vi "CLSUIP_UnlockNewVI.vi"(8 "error in (no error)":errorcluster, 11 "VIRetooler":refnum<class "VIRetooler.lvclass">) -> (0 "error out":errorcluster)   [LabVIEW 2021, in "MemberVICreation.lvlib" / "VIRetooler.lvclass"]
uses:
  <resource>/Framework/Providers/LVClassLibrary/NewAccessors/VIRetooler/VIRetooler.lvclass
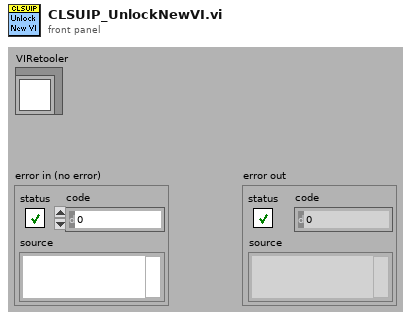
[diagram p1: front panel]
types:
  T1 = enum32{"invalid lock state", "Not Locked", "Locked (No Password)", "Password-protected"}
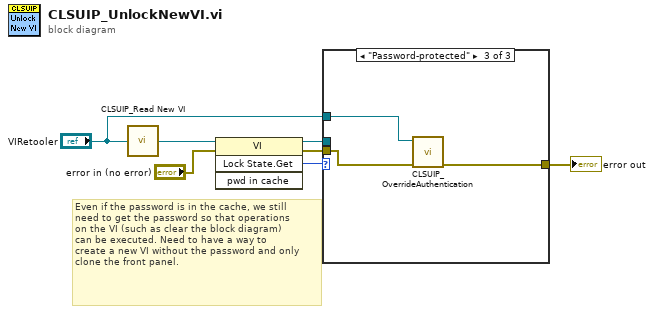
[diagram p0: block diagram]
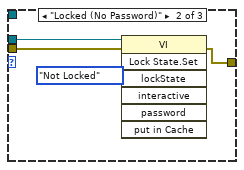
[diagram p3: hidden frame]
diagram:
  # "Even if the password is in the cache, we still\nneed to get the password so that operations\non the VI (such as clear the block diagram)\ncan be executed. Need to have a way to\ncreate a new VI without the password and only\nclone the front panel."
  n1 = call <resource>:"CLSUIP_Read New VI.vi"("VIRetooler.lvclass in"="VIRetooler") -> ("New VI"=w3:refnum<vi>)
  n2 = invoke class="VI" method="Lock State.Get"(reference=w3, error in="error in (no error)") -> (reference out=w1:refnum<vi>, error out=w5:errorcluster, "Get Lock State"=w6:T1)  [unwired: 2 in, 1 out]
  n3 = case shown="\"Password-protected\"" w6 {
    tunnel: w5 -> [w8 w12 w15]
    tunnel: [w8 w10 w14] -> w4
    tunnel: "VIRetooler" -> [_ _ w13]
    tunnel: w1 -> [_ w9 _]
    frame "Not Locked", Default {
    }
    frame "Locked (No Password)" {
      n4 = invoke class="VI" method="Lock State.Set"(reference=w9, error in=w12, "lockState"=T1."Not Locked" ("Lock State")) -> (error out=w10:errorcluster)  [unwired: 4 in, 6 out]
    }
    frame "Password-protected" {
      n5 = call <resource>:"CLSUIP_OverrideAuthentication.vi"("error in (no error)"=w15, "VIRetooler"=w13) -> ("error out"=w14:errorcluster)  [unwired: 1 in, 8 out]
    }
  }
  "error out" <- w4
